vi "Example.vi"() -> ()   [LabVIEW 2018]
uses:
  Data Def/Kikusui PLZ-Setting.ctl
panel:
  in  "Tracer":bool
  in  "Apply":bool
  in  "Value":dbl
  in  "Operation Mode":enum16{"CC", "CV", "CP"}(ring)
  out "Input?":bool
  in  "Stop Load":bool
  in  "Apply Load":bool
  out "Chart":T1(graph)
  out "Stop?":bool
  in  "Kikusui PLZ Setting In":T2={"VISA Resource Name"="USB0::0x0B3E::0x1020::YJ002260::INSTR", "Baud Rate"=19200, "Stop Bits"=20, "Wait For Read(ms)"=10} {"Stop Bits" items=["1.0"=10, "2.0"=20]; "Baud Rate" items=["2400"=2400, "4800"=4800, "9600"=9600, "19200"=19200]}
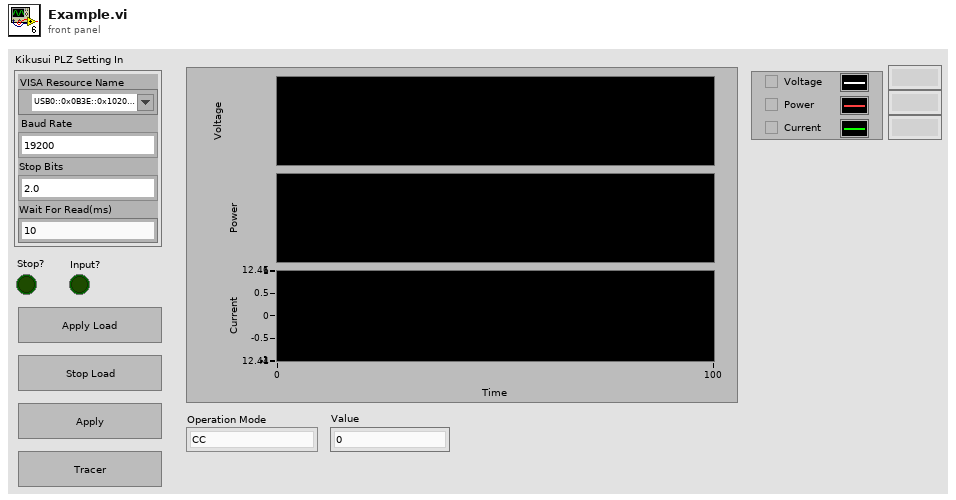
[diagram p1: front panel]
types:
  T1 = cluster{"Voltage (Volts)":dbl, "Power (Watts)":dbl, "Current (Amps)":dbl}
  T2 = typedef "Kikusui PLZ-Setting.ctl" = cluster{"VISA Resource Name":refnum<visa-resource-name>, "Baud Rate":u32, "Stop Bits":u16, "Wait For Read(ms)":u32}
  T3 = typedef "Kikusui PLZ-Measurement Data.ctl" = cluster{"Current (Amps)":dbl, "Power (Watts)":dbl, "Voltage (Volts)":dbl, "Elapsed Time (Sec) ":dbl}
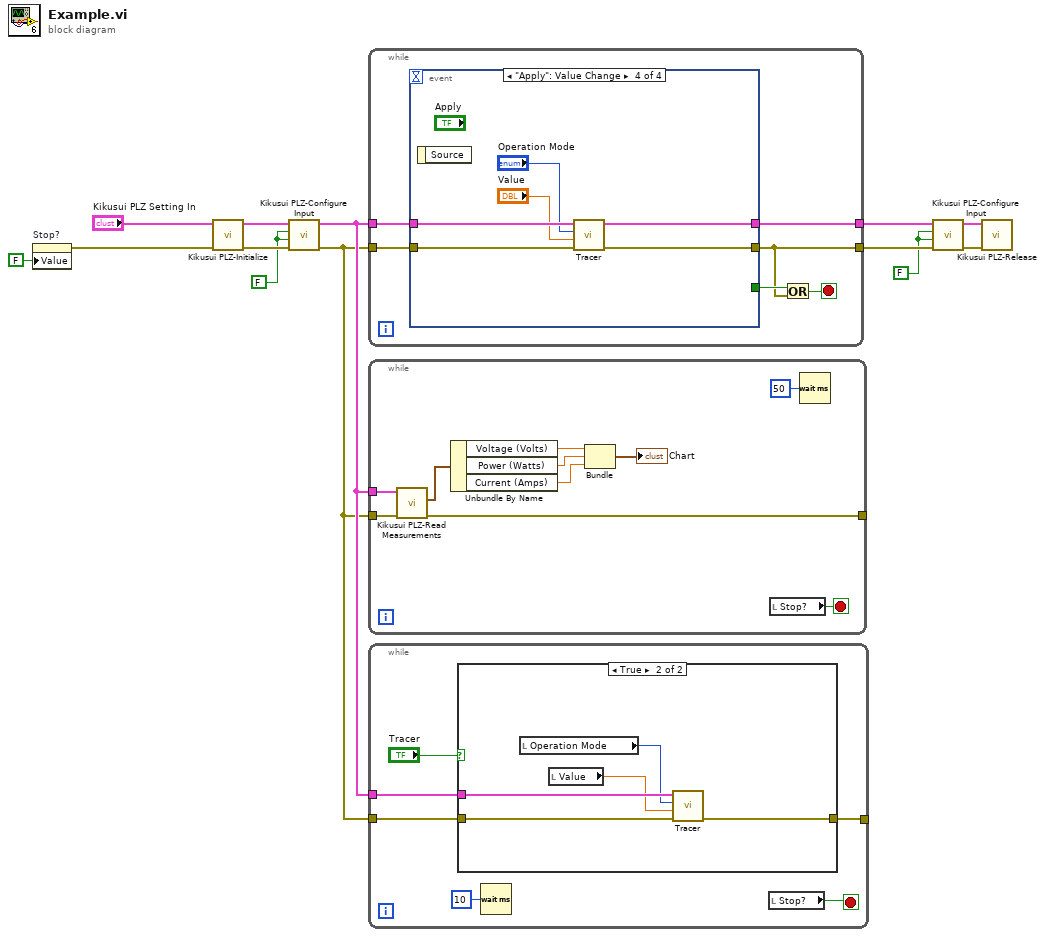
[diagram p0: block diagram]
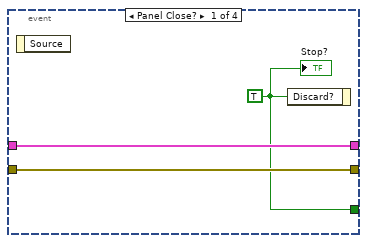
[diagram p3: hidden frame]
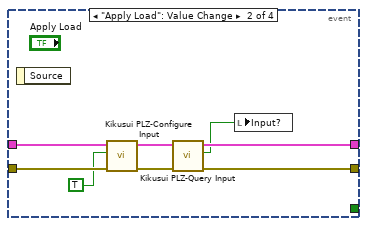
[diagram p4: hidden frame]
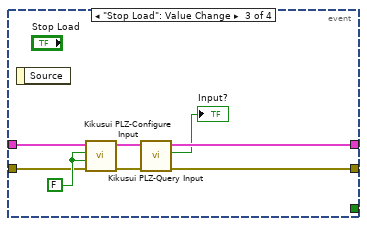
[diagram p5: hidden frame]
diagram:
  w5 = FALSE ("Enable Input")
  w10 = FALSE ("Enable Input")
  n1 = property on="Stop?" class="Bool (strict)"("Value"=FALSE ("Stop?")) -> (error out=w4:errorcluster)  [unwired: 2 in, 1 out]
  n2 = call "Kikusui PLZ-Initialize.vi"("error in"=w4, "Kikusui PLZ Setting In"="Kikusui PLZ Setting In") -> ("error out"=w11:errorcluster, "Kikusui PLZ Setting Out"=w12:T2)  [unwired: 8 in]
  n3 = call "Kikusui PLZ-Configure Input.vi"("error in"=w11, "Enable Input Short"=w10, "Enable Input"=w10, "Kikusui PLZ Setting In"=w12) -> ("error out"=w1:errorcluster, "Kikusui PLZ Setting Out"=w2:T2)  [unwired: 6 in]
  n4 = while {
    tunnel: w2 -> [w18]
    tunnel: w1 -> [w19]
    tunnel: [w16] -> w8
    tunnel: [w14] -> w9
    stop <- w15 stop-if-true
    n5 = event shown="[3] \"Apply\": Value Change" {
      selector: _ -> [_ _ _ _]
      dyn-events: _ -> [_ _ _ _]
      timeout: _ -> [_ _ _ _]
      tunnel: w19 -> [w22 w29 w36 w43]
      tunnel: w18 -> [w21 w30 w37 w44]
      tunnel: [w22 w25 w33 w42] -> w16
      tunnel: [w20 _ _ _] -> w17
      tunnel: [w21 w24 w32 w41] -> w14
      event Panel Close? {
        w20 = TRUE ("Discard?")
        n6 = event-data() -> ()  [unwired: 1 in, 1 out]
        n7 = event-data("Discard?"=w20) -> ()  [unwired: 1 in, 1 out]
        "Stop?" <- w20
      }
      event "Apply Load": Value Change {
        n8 = event-data() -> ()  [unwired: 1 in, 1 out]
        n9 = call "Kikusui PLZ-Configure Input.vi"("error in"=w29, "Enable Input"=TRUE, "Kikusui PLZ Setting In"=w30) -> ("error out"=w26:errorcluster, "Kikusui PLZ Setting Out"=w27:T2)  [unwired: 7 in]
        n10 = call "Kikusui PLZ-Query Input.vi"("error in"=w26, "Kikusui PLZ Setting In"=w27) -> ("error out"=w25:errorcluster, "Input?"=w23:bool, "Kikusui PLZ Setting Out"=w24:T2)  [unwired: 7 in]
        n11 = local write "Input?"(w23) -> ()
      }
      event "Stop Load": Value Change {
        w38 = FALSE ("Enable Input")
        n12 = event-data() -> ()  [unwired: 1 in, 1 out]
        n13 = call "Kikusui PLZ-Configure Input.vi"("error in"=w36, "Enable Input Short"=w38, "Enable Input"=w38, "Kikusui PLZ Setting In"=w37) -> ("error out"=w34:errorcluster, "Kikusui PLZ Setting Out"=w35:T2)  [unwired: 6 in]
        n14 = call "Kikusui PLZ-Query Input.vi"("error in"=w34, "Kikusui PLZ Setting In"=w35) -> ("error out"=w33:errorcluster, "Input?"=→"Input?":bool, "Kikusui PLZ Setting Out"=w32:T2)  [unwired: 7 in]
      }
      event "Apply": Value Change {
        n15 = event-data() -> ()  [unwired: 1 in, 1 out]
        n16 = call "Tracer.vi"("error in"=w43, "Value"="Value", "Operation Mode"="Operation Mode", "Kikusui PLZ Setting In"=w44) -> ("error out"=w42:errorcluster, "Kikusui PLZ Setting Out"=w41:T2)  [unwired: 6 in]
      }
    }
    n17 = Or(x=w17, y=w16) -> (x .or. y?=w15:bool)
  }
  n18 = while {
    tunnel: w2 -> [w52]
    tunnel: w1 -> [w53]
    tunnel: [w47] -> _
    stop <- w54 stop-if-true
    n19 = call "Kikusui PLZ-Read Measurements.vi"("error in"=w53, "Kikusui PLZ Setting In"=w52) -> ("error out"=w47:errorcluster, "Measurement Data"=w51:T3)  [unwired: 7 in, 1 out]
    n20 = Unbundle By Name(w51) -> ("Voltage (Volts)"=w50:dbl, "Power (Watts)"=w49:dbl, "Current (Amps)"=w48:dbl)
    n21 = Bundle("Voltage (Volts)"=w50, "Power (Watts)"=w49, "Current (Amps)"=w48) -> (→"Chart":T1)  [unwired: 1 in]
    n22 = local read "Stop?"() -> (w54:bool)
    n23 = Wait (ms)(milliseconds to wait=u32 50) -> ()  [unwired: 1 out]
  }
  n24 = while {
    tunnel: w2 -> [w57]
    tunnel: w1 -> [w56]
    tunnel: [w55] -> _
    stop <- w60 stop-if-true
    n25 = case shown="True" "Tracer" {
      tunnel: w57 -> [_ w66]
      tunnel: w56 -> [w61 w65]
      tunnel: [w61 w64] -> w55
      frame False {
      }
      frame True {
        n26 = local read "Operation Mode"() -> (w63:enum16{"CC", "CV", "CP"})
        n27 = local read "Value"() -> (w62:dbl)
        n28 = call "Tracer.vi"("error in"=w65, "Value"=w62, "Operation Mode"=w63, "Kikusui PLZ Setting In"=w66) -> ("error out"=w64:errorcluster)  [unwired: 6 in, 1 out]
      }
    }
    n29 = Wait (ms)(milliseconds to wait=u32 10) -> ()  [unwired: 1 out]
    n30 = local read "Stop?"() -> (w60:bool)
  }
  n31 = call "Kikusui PLZ-Configure Input.vi"("error in"=w8, "Enable Input Short"=w5, "Enable Input"=w5, "Kikusui PLZ Setting In"=w9) -> ("error out"=w6:errorcluster, "Kikusui PLZ Setting Out"=w7:T2)  [unwired: 6 in]
  n32 = call "Kikusui PLZ-Release.vi"("error in"=w6, "Kikusui PLZ Setting"=w7) -> ()  [unwired: 9 in, 1 out]
